vi "_17_Sample_qsns_05[26].vi"() -> ()   [LabVIEW 2020]
panel:
  out "x/y":dbl
  in  "stop":bool
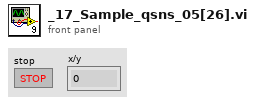
[diagram p1: front panel]
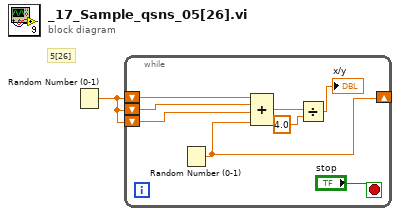
[diagram p0: block diagram]
diagram:
  # "5[26]"
  n1 = Random Number (0-1)() -> (number: 0 to 1=w1:dbl)
  n2 = while {
    shift-right: [w6] -> _
    shift-left: w1 -> [w9]
    shift-left: w1 -> [w8]
    shift-left: w1 -> [w7]
    stop <- "stop" stop-if-true
    n3 = Random Number (0-1)() -> (number: 0 to 1=w6:dbl)
    n4 = Compound Arithmetic op=ADD(w9, w8, w7, w6) -> (w5:dbl)
    n5 = Divide(x=w5, y=4.0) -> (x/y=→"x/y":dbl)
  }
